vi "路径分析-8.6.vi"(8 "第二个文件夹":string="EV01", 9 "第一个文件夹":string="主板监控数据", 11 "输入路径":path) -> (3 "输出路径":path)   [LabVIEW 2013]
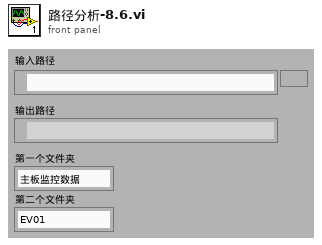
[diagram p1: front panel]
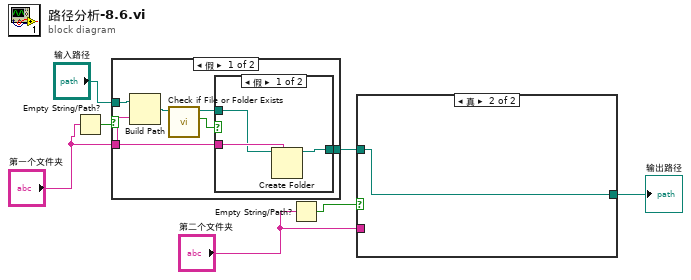
[diagram p0: block diagram]
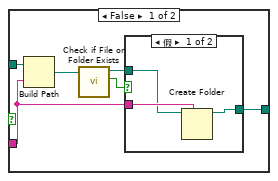
[diagram p4: hidden frame]
diagram:
  n1 = Empty String/Path?(string/path="第一个文件夹") -> (empty?=w1:bool)
  n2 = case shown="假" w1 {
    tunnel: "输入路径" -> [w13 w18]
    tunnel: "第一个文件夹" -> [w10 _]
    tunnel: [w8 w18] -> w6
    frame False {
      n3 = Build Path(base path=w13, name or relative path=w10) -> (appended path=w12:path)
      n4 = call <vilib>:"Check if File or Folder Exists.vi"("path"=w12) -> ("file or folder exists?"=w11:bool, "dup path"=w9:path)  [unwired: 1 in, 8 out]
      n5 = case shown="假" w11 {
        tunnel: w10 -> [w16 _]
        tunnel: w9 -> [w15 w17]
        tunnel: [w14 w17] -> w8
        frame False {
          n6 = Create Folder(prompt (Create Folder)=w16, path (use dialog)=w15) -> (created path=w14:path)  [unwired: 1 in, 2 out]
        }
        frame True {
        }
      }
    }
    frame True {
    }
  }
  n7 = Empty String/Path?(string/path="第二个文件夹") -> (empty?=w3:bool)
  n8 = case shown="真" w3 {
    tunnel: w6 -> [w24 w29]
    tunnel: "第二个文件夹" -> [w20 _]
    tunnel: [w19 w29] -> w5
    frame False {
      n9 = Build Path(base path=w24, name or relative path=w20) -> (appended path=w21:path)
      n10 = call <vilib>:"Check if File or Folder Exists.vi"("path"=w21) -> ("file or folder exists?"=w22:bool, "dup path"=w23:path)  [unwired: 1 in, 8 out]
      n11 = case shown="假" w22 {
        tunnel: w20 -> [w27 _]
        tunnel: w23 -> [w26 w28]
        tunnel: [w25 w28] -> w19
        frame False {
          n12 = Create Folder(prompt (Create Folder)=w27, path (use dialog)=w26) -> (created path=w25:path)  [unwired: 1 in, 2 out]
        }
        frame True {
        }
      }
    }
    frame True {
    }
  }
  "输出路径" <- w5
